vi "Get Log File Settings.vi"(8 "error in (no error)":errorcluster, 11 "File Ref in":T1 format="%.0x") -> (0 "error out":errorcluster, 1 "File Path - RT Targets":path, 2 "File Path - Windows":path, 3 "File Ref out":T1 format="%.0x", 4 "Ovewrite File If Exists?":bool)   [LabVIEW 2020, in "Telemetry System Explorer.lvlib"]
uses:
  Telemetry System Explorer.lvlib
  <vilib>/NI VeriStand/Custom Device API/Custom Device Item Ref.ctl
  Shared/Constants.vi
  <vilib>/NI VeriStand/Custom Device API/Get Item Property (Boolean).vi
  <vilib>/NI VeriStand/Custom Device API/Custom Device API.lvlib
  Shared/Telemetry Shared.lvlib
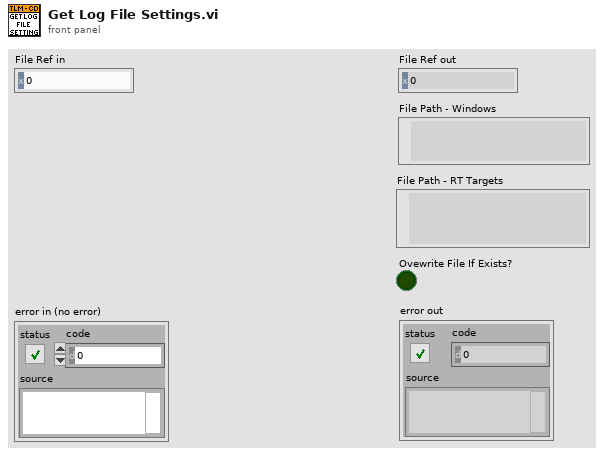
[diagram p1: front panel]
types:
  T1 = typedef "Custom Device API.lvlib/Custom Device Item Ref.ctl" = u64
  T2 = enum16{"PharLap", "VxWorks", "Windows", "Linux_32_ARM", "Linux_x64"}
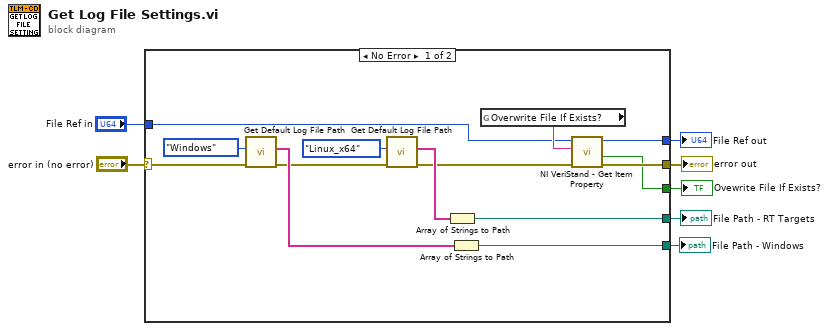
[diagram p0: block diagram]
diagram:
  n1 = case shown="No Error" "error in (no error)" {
    selector: "error in (no error)" -> [w8 w23]
    tunnel: [w20 _] -> w7
    tunnel: [w19 w22] -> w6
    tunnel: [w18 w23] -> w5
    tunnel: [w17 _] -> w4
    tunnel: "File Ref in" -> [w16 w22]
    tunnel: [w12 _] -> w2
    frame No Error {
      n2 = call "Get Default Log File Path.vi"("error in"=w8, "Target Type"=T2."Windows") -> ("error out"=w10:errorcluster, "Log File Path String Array"=w14:string[])  [unwired: 8 in]
      n3 = call "Get Default Log File Path.vi"("error in"=w10, "Target Type"=T2."Linux_x64") -> ("error out"=w9:errorcluster, "Log File Path String Array"=w11:string[])  [unwired: 8 in]
      n4 = Array of Strings to Path(0:w11) -> (2:w12:path)  [unwired: 1 in]
      n5 = Array of Strings to Path(0:w14) -> (2:w20:path)  [unwired: 1 in]
      n6 = global read "Constants.vi" "Overwrite File If Exists?"() -> (w21:string)
      n7 = call-poly <vilib>:"NI VeriStand - Get Item Property.vi"("error in (no error)"=w9, "Property Name"=w21, "Item Ref in"=w16) -> ("error out"=w18:errorcluster, "Value"=w17:bool, "Item Ref out"=w19:T1)  [unwired: 1 in, 5 out]
    }
    frame Error {
    }
  }
  "error out" <- w5
  "File Path - Windows" <- w7
  "File Ref out" <- w6
  "Ovewrite File If Exists?" <- w4
  "File Path - RT Targets" <- w2
